vi "Set Standard.vi"(8 "error in (no error)":errorcluster, 11 "Servo MSMT in":refnum<class "Servo MSMT.lvclass">) -> (0 "error out":errorcluster, 3 "Servo MSMT out":refnum<class "Servo MSMT.lvclass">)   [LabVIEW 2018, in "Servo MSMT.lvlib" / "Servo MSMT.lvclass"]
uses:
  Servo MSMT.lvclass
  C:/Sequence Automation/Plugins/Measurement Interface.lvlibp/Measurement Interface.lvclass
  Plugins/Measurement Interface.lvlibp/Private Methods/Measurement Definition Entry/Read Measurement Definition Entry.vi
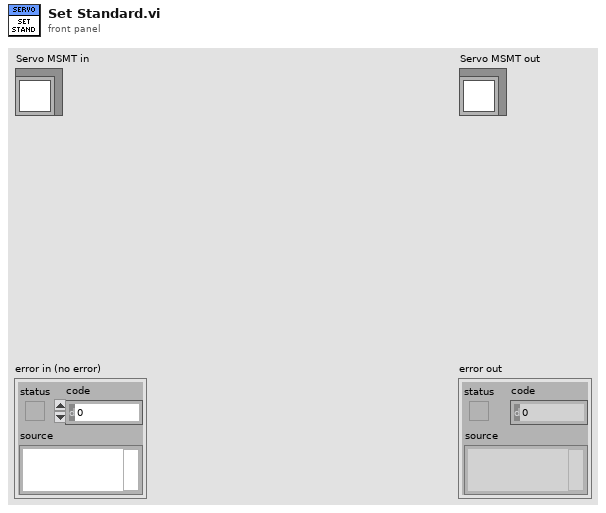
[diagram p1: front panel]
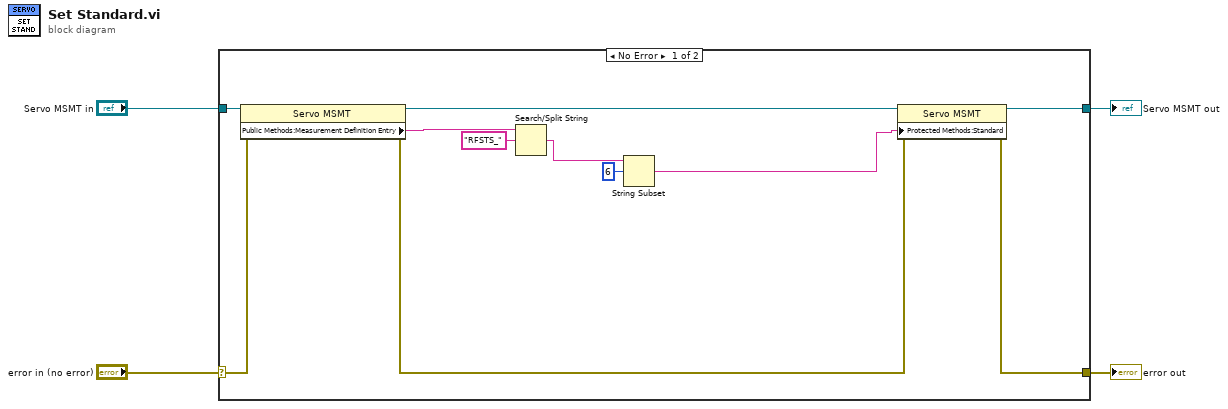
[diagram p0: block diagram]
diagram:
  n1 = case shown="No Error" "error in (no error)" {
    selector: "error in (no error)" -> [w15 w17]
    tunnel: [w10 w17] -> w3
    tunnel: [w8 w16] -> w1
    tunnel: "Servo MSMT in" -> [w13 w16]
    frame No Error {
      n2 = property class="Servo MSMT"(reference=w13, error in=w15) -> (reference out=w9:refnum<class "Servo MSMT.lvclass">, error out=w14:errorcluster, "Public Methods:Measurement Definition Entry"=w12:string)
      n3 = Search/Split String(string=w12, search string/char (-)="RFSTS_") -> (match + rest of string=w7:string)  [unwired: 1 in, 2 out]
      n4 = String Subset(string=w7, offset (0)=6) -> (substring=w5:string)  [unwired: 1 in]
      n5 = property class="Servo MSMT"(reference=w9, error in=w14, "Protected Methods:Standard"=w5) -> (reference out=w8:refnum<class "Servo MSMT.lvclass">, error out=w10:errorcluster)
    }
    frame Error {
    }
  }
  "error out" <- w3
  "Servo MSMT out" <- w1
